vi "Check Shield.vi"(7 "Packed refs":T1, 8 "error in (no error)":errorcluster, 11 "Board Game in":refnum<class "Board Game.lvclass">) -> (0 "error out":errorcluster, 3 "Board Game out":refnum<class "Board Game.lvclass">)   [LabVIEW 2021, in "Board Game.lvclass"]
uses:
  Board Game.lvclass
  Application/Packed Refs.ctl
  GameEl_class/private/Enum Direction.ctl
  LVApp/Modules/Sound Manager/Typedefs/Sound Effects.ctl
  Board Game.lvclass/Board Game.ctl
  Snake_class/Snake.lvclass/Snake.ctl
  GameEl_class/GameEl.lvclass/GameEl.ctl
  Shield/Shield.lvclass/Shield.ctl
  <vilib>/numeric/Random Number (Range) U64.vi
  Shield/Read Shield Count.vi
  GameEl_class/Read Visible.vi
  GameEl_class/Read position.vi
  Snake_class/Read Star.vi
  Snake_class/Read Snake Head.vi
  <vilib>/numeric/sub_Random U32.vi
  Shield/Shield.lvclass
  C:/Users/poche/Programs/LabVIEW/imposible snake/GameEl_class/GameEl.lvclass
  Snake_class/Snake.lvclass
  GameEl_class/GameEl.lvclass
  Application/Application.lvclass
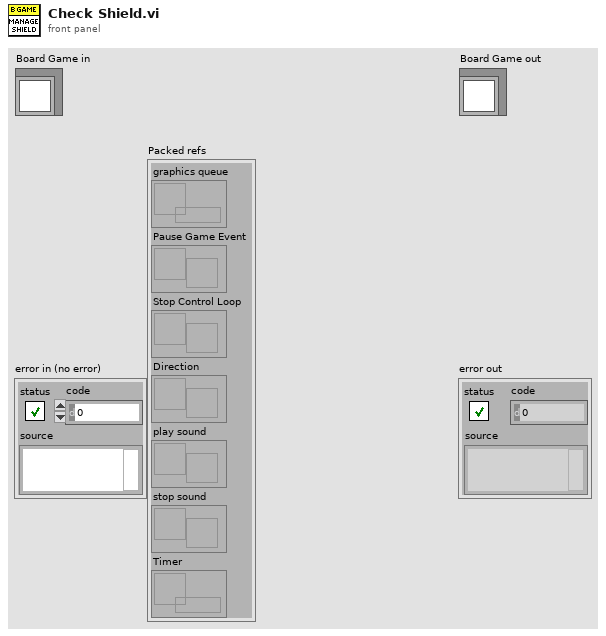
[diagram p1: front panel]
types:
  T1 = typedef "Application.lvclass/Packed Refs.ctl" = cluster{"graphics queue":refnum<queue>, "Pause Game Event":refnum<user-event>, "Stop Control Loop":refnum<user-event>, "Direction":refnum<notifier>, "play sound":refnum<user-event>, "stop sound":refnum<user-event>, "Timer":refnum<data-value>}
  T2 = typedef "Sound Effects.ctl" = enum16{"Bomb In", "Bomb Out", "Bomb Touched", "Game Over", "Victory", "Eat", "10 Fruits", "Eat2", "Eat3", "Eat4", "MaxShield", "Shield", "10p", "Grape In", "Grape Out", "20p", "30p", "40p", "50p", "60p", "70p", "80p", "90p", "100p", "All shields cracked", "Mouse In", "Mouse Out", "Mouse Eaten", "Grape Eaten", "States Recover", "Broken Shield", "Bonus", "Happy Time", "explode", "Game over musica", "Back Music", "Shield Catch", "Evil lough", "Cricket In", "Cricket eaten", "Lets Go", "Jump1", "Jump2", "Jump3", "Unstoppable", "Troll Music", "winner"}
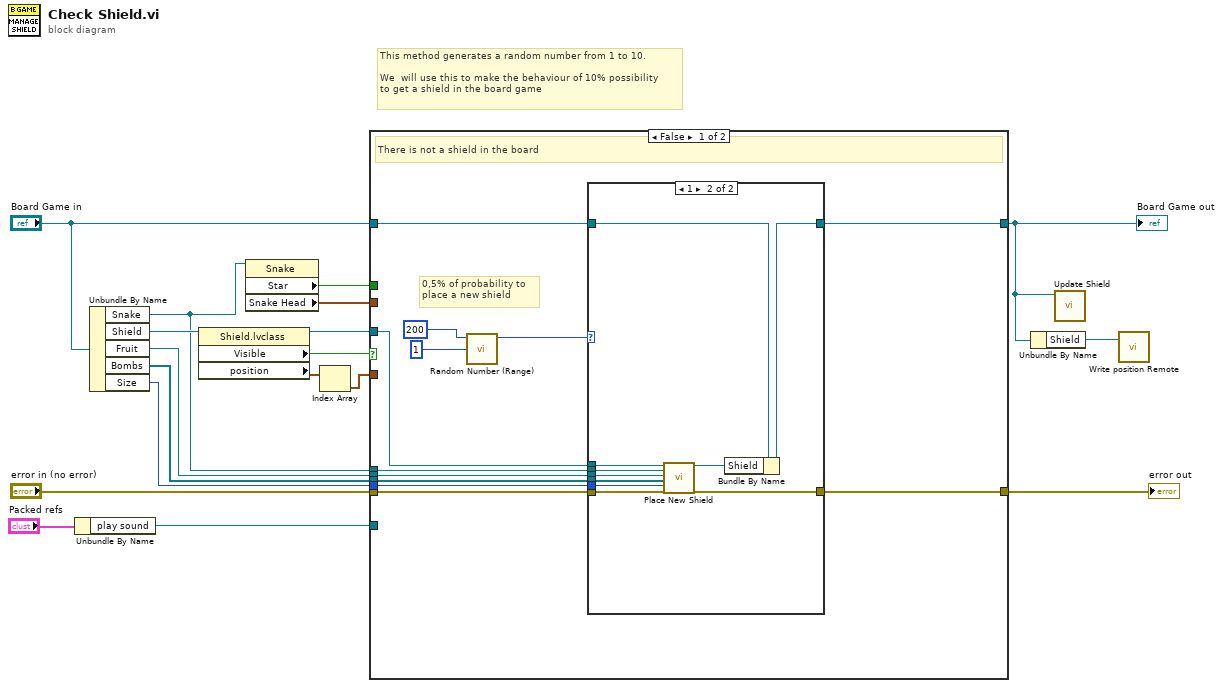
[diagram p0: block diagram]
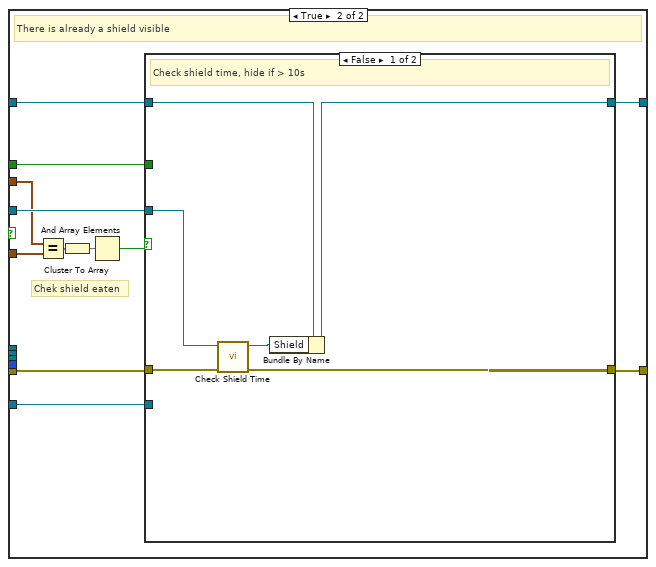
[diagram p3: hidden frame]
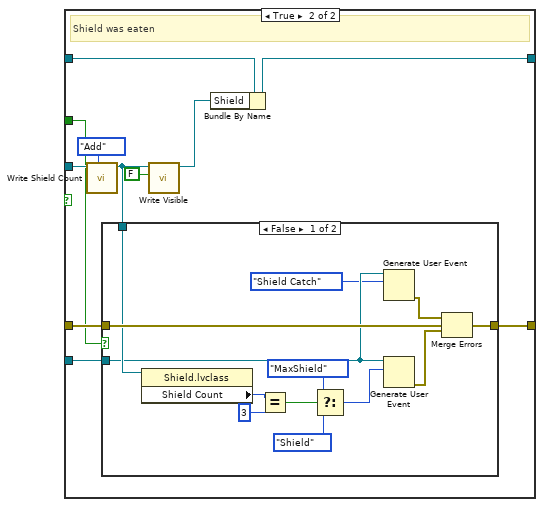
[diagram p4: hidden frame]
diagram:
  # "This method generates a random number from 1 to 10. \n\nWe  will use this to make the behaviour of 10% possibility\nto get a shield in the board game"
  n1 = Unbundle By Name("Packed refs") -> ("play sound"=w2:refnum<user-event>)
  n2 = Unbundle By Name("Board Game in") -> ("Snake"=w10:refnum<class "Snake.lvclass">, "Shield"=w18:refnum<class "Shield.lvclass">, "Fruit"=w9:refnum<class "Fruit.lvclass">, "Bombs"=w8:refnum<class "Bomb.lvclass">[], "Size"=w7:u16)
  n3 = property class="Shield.lvclass"(reference=w18) -> (reference out=w13:refnum<class "Shield.lvclass">, "Visible"=w14:bool, "position"=w12:cluster{"x":dbl, "y":dbl}[])  [unwired: 1 in, 1 out]
  n4 = property class="Snake"(reference=w10) -> ("Star"=w1:bool, "Snake Head"=w11:cluster{"x":dbl, "y":dbl})  [unwired: 1 in, 2 out]
  n5 = Index Array(array=w12) -> (element=w6:cluster{"x":dbl, "y":dbl})  [unwired: 1 in]
  n6 = case shown="False" w14 {
    tunnel: "error in (no error)" -> [w28 w49]
    tunnel: [w27 w48] -> w16
    tunnel: "Board Game in" -> [w26 w47]
    tunnel: [w25 w46] -> w5
    tunnel: w13 -> [w23 w54]
    tunnel: w6 -> [_ w53]
    tunnel: w11 -> [_ w52]
    tunnel: w10 -> [w22 _]
    tunnel: w9 -> [w21 _]
    tunnel: w8 -> [w20 _]
    tunnel: w7 -> [w19 _]
    tunnel: w2 -> [_ w44]
    tunnel: w1 -> [_ w43]
    frame False {
      # "0,5% of probability to \nplace a new shield"
      # "There is not a shield in the board"
      n7 = call-poly <vilib>:"Random Number (Range).vi"("lower bound (0)"=u64 1, "upper bound (100)"=u64 200) -> ("number"=w24:u64)  [unwired: 9 in]
      n8 = case shown="1" w24 {
        tunnel: w28 -> [w31 w42]
        tunnel: [w31 w41] -> w27
        tunnel: w26 -> [w32 w40]
        tunnel: [w32 w34] -> w25
        tunnel: w23 -> [_ w39]
        tunnel: w22 -> [_ w38]
        tunnel: w21 -> [_ w37]
        tunnel: w20 -> [_ w36]
        tunnel: w19 -> [_ w35]
        frame 0, Default {
        }
        frame 1 {
          n9 = call "Place New Shield.vi"("Shield in"=w39, "Snake"=w38, "Fruit in"=w37, "Bomb"=w36, "B Game Size"=w35, "error in (no error)"=w42) -> ("Shield out"=w33:refnum<class "Shield.lvclass">, "error out"=w41:errorcluster)  [unwired: 12 in]
          n10 = Bundle By Name(cluster=w40, "Shield"=w33) -> (w34:refnum<class "Board Game.lvclass">)
        }
      }
    }
    frame True {
      # "Chek shield eaten"
      # "There is already a shield visible"
      n11 = Equal?(x=w52, y=w53) -> (x = y?=w50:cluster{"x":bool, "y":bool})
      n12 = Cluster To Array(cluster=w50) -> (array=w51:bool[])
      n13 = And Array Elements(Boolean array=w51) -> (logical AND=w45:bool)
      n14 = case shown="False" w45 {
        tunnel: w54 -> [w59 w70]
        tunnel: w49 -> [w60 w71]
        tunnel: [w55 w62] -> w48
        tunnel: w47 -> [w58 w68]
        tunnel: [w57 w67] -> w46
        tunnel: w44 -> [_ w63]
        tunnel: w43 -> [_ w61]
        frame False {
          # "Check shield time, hide if > 10s"
          n15 = call "Check Shield Time.vi"("error in (no error)"=w60, "Shield in"=w59) -> ("error out"=w55:errorcluster, "Shield out"=w56:refnum<class "Shield.lvclass">)  [unwired: 8 in]
          n16 = Bundle By Name(cluster=w58, "Shield"=w56) -> (w57:refnum<class "Board Game.lvclass">)
        }
        frame True {
          # "Shield was eaten"
          n17 = call "Write Shield Count.vi"("function"=enum16{"Add", "Subtract"}."Add", "Shield in"=w70) -> ("Shield out"=w66:refnum<class "Shield.lvclass">)  [unwired: 8 in, 1 out]
          n18 = case shown="False" w61 {
            tunnel: w71 -> [w84 w85]
            tunnel: w66 -> [w83 _]
            tunnel: w63 -> [w76 _]
            tunnel: [w74 w85] -> w62
            frame False {
              n19 = property class="Shield.lvclass"(reference=w83) -> ("Shield Count"=w82:u8)  [unwired: 1 in, 2 out]
              n20 = Equal?(x=w82, y=u8 3) -> (x = y?=w80:bool)
              n21 = Select(t=Sound_Effects."MaxShield" ("event data"), s=w80, f=Sound_Effects."Shield" ("event data")) -> (s? t:f=w77:T2)
              n22 = Generate User Event(user event=w76, event data cluster=Sound_Effects."Shield Catch" ("event data")) -> (error out=w73:errorcluster)  [unwired: 2 in, 1 out]
              n23 = Generate User Event(user event=w76, event data cluster=w77) -> (error out=w72:errorcluster)  [unwired: 2 in, 1 out]
              n24 = Merge Errors(w73, w84, w72) -> (w74:errorcluster)
            }
            frame True {
            }
          }
          n25 = call "Write Visible.vi"("Visible"=FALSE, "GameEl in"=w66) -> ("GameEl out"=w65:refnum<class "Shield.lvclass">)  [unwired: 8 in, 1 out]
          n26 = Bundle By Name(cluster=w68, "Shield"=w65) -> (w67:refnum<class "Board Game.lvclass">)
        }
      }
    }
  }
  "error out" <- w16
  "Board Game out" <- w5
  n27 = Unbundle By Name(w5) -> ("Shield"=w4:refnum<class "Shield.lvclass">)
  n28 = call "Update Shield.vi"("Board Game in"=w5) -> ()  [unwired: 11 in]
  n29 = call "Write position Remote.vi"("GameEl in"=w4) -> ()  [unwired: 10 in, 1 out]
